vi "test_generic.vi"() -> ()   [LabVIEW 2017, in "GenericDAQ.lvclass"]
uses:
  GenericDAQ.lvclass
  Clock/GenericClock/GenericClock/GenericClock.lvclass
  common/classes/GenericComponent/GenericComponent/GenericComponent.lvclass
  main/labview_source/type_definitions/clusters/controls_refs.ctl
  common/classes/ErrorController/ErrorController/ErrorController.lvclass
  common/classes/GenericToplevelComponent/GenericToplevelComponent/common_trigger_enum.ctl
  common/classes/GenericToplevelComponent/GenericToplevelComponent/GenericToplevelComponent.lvclass
  main/labview_source/type_definitions/enumerations/run_mode_enum.ctl
panel:
  out "error handler loaded?":bool
  in  "toggleAcquisitionButton":bool
  in  "continuous?":bool
  in  "samples to read":i32=1000000000
  in  "frequency":dbl[unit]=40000.0
  in  "createClockButton":bool
  in  "createDAQButton":bool
  out "error out":errorcluster
  in  "stopProgramButton":bool
  # "Test Suite for GenericDAQ"
  # "How to use this Test Suite\n\n1. Choose DAQ compoment and select configuration. \n2. Create and send DAQ component.\n3. Choose Clock component and select configuration.\n4. Create Clock component.\n5. Start Clock."
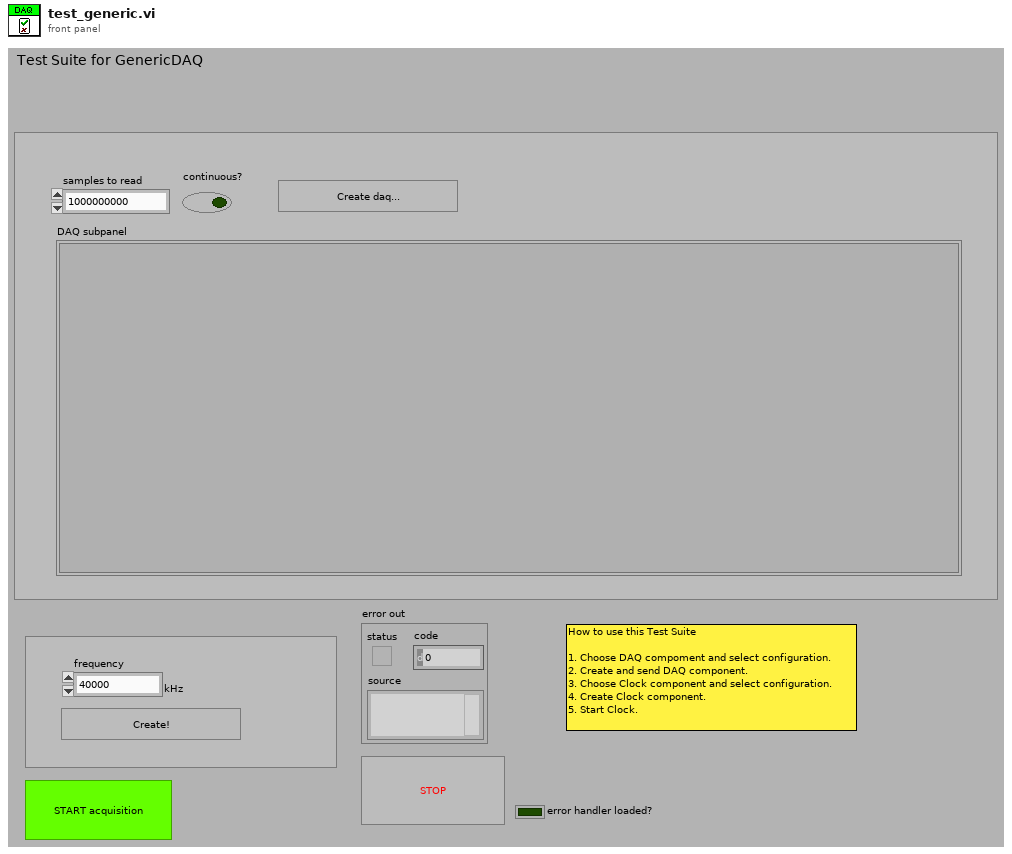
[diagram p1: front panel]
types:
  T1 = typedef "controls_refs.ctl" = cluster{"buttons":cluster{"start_focus":refnum<vi>, "start_single_sweep":refnum<vi>, "start_experiment":refnum<vi>, "save":refnum<vi>, "exit":refnum<vi>}, "tabs":cluster{"main":refnum<vi>, "settings":refnum<vi>}, "subpanels":cluster{"imagingMode":refnum<vi>, "scanHead":refnum<vi>, "display":refnum<vi>, "experimentController":refnum<vi>, "instrument":refnum<vi>, "stage":refnum<vi>, "stimulator":refnum<vi>, "dataCollection":refnum<vi>, "analyser":refnum<vi>, "daq":refnum<vi>, "imageAssembler":refnum<vi>}, "drop-downs":cluster{"imagingMode":refnum<vi>, "experimentalController":refnum<vi>, "objective":refnum<vi>}, "status lights":cluster{"experimentController":refnum<vi>, "imagingMode":refnum<vi>, "scanHead":refnum<vi>, "daq":refnum<vi>, "imageAssembler":refnum<vi>, "dataCollection":refnum<vi>, "display":refnum<vi>, "analyser":refnum<vi>, "stage":refnum<vi>, "stimulator":refnum<vi>, "instrument":refnum<vi>}, "message":refnum<vi>, "stimulator enabled?":refnum<vi>, "saving":cluster{"data folder path":refnum<vi>, "file base name":refnum<vi>, "notebook":refnum<vi>}, "progress bar":refnum<vi>, "update icon":refnum<vi>, "title":refnum<vi>, "main vi":refnum<vi>, "user":refnum<vi>}
  T2 = typedef "run_mode_enum.ctl" = enum16{"focus mode", "single sweep mode", "experiment mode"}
  T3 = typedef "GenericToplevelComponent.lvclass/common_trigger_enum.ctl" = enum16{"NULL", "initialise", "terminate", "fetch command", "fetch data", "attach observer", "register as observer", "detach observer", "acknowledge", "start", "stop", "sweep started", "sweep finished", "experiment started", "experiment stopped"}
  T4 = typedef "XComponentSpecification.xctl/data.ctl" = cluster{"class path":string, "configuration":string, "label":string, "settings name":string}
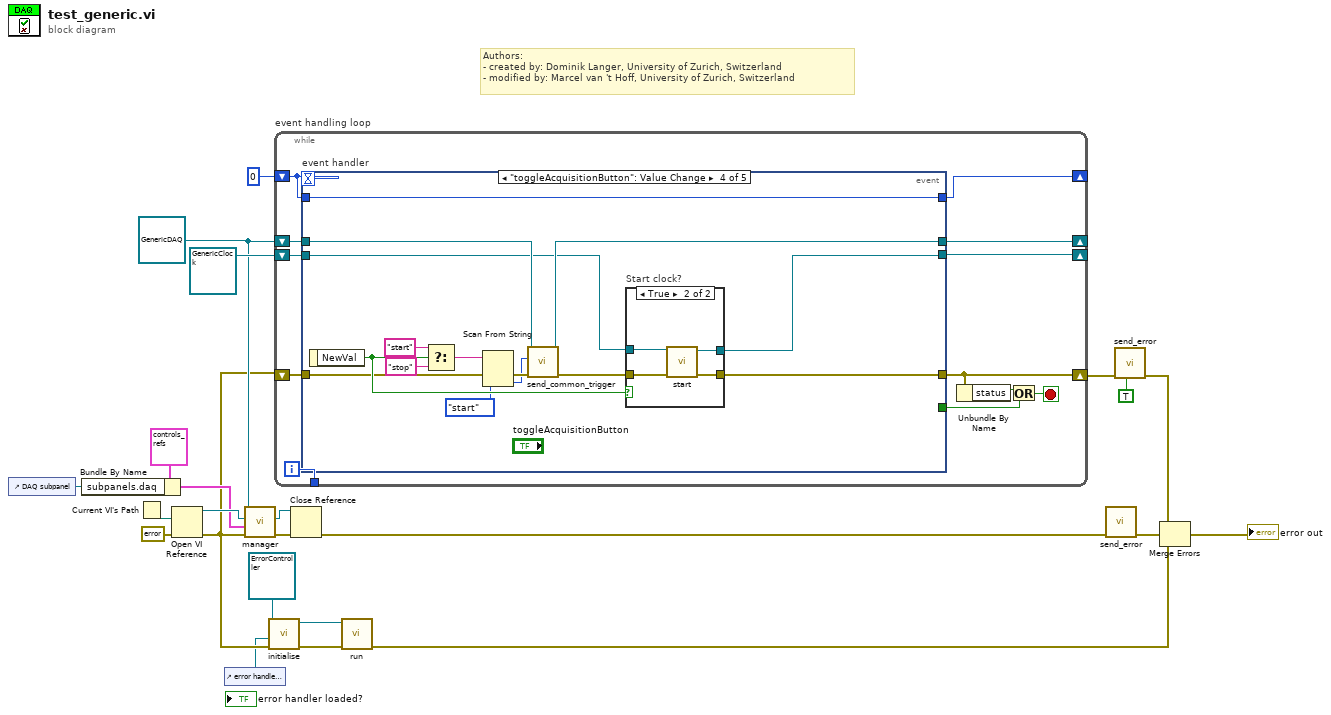
[diagram p0: block diagram]
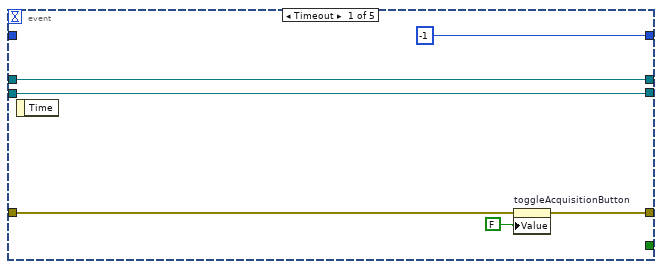
[diagram p2: hidden frame]
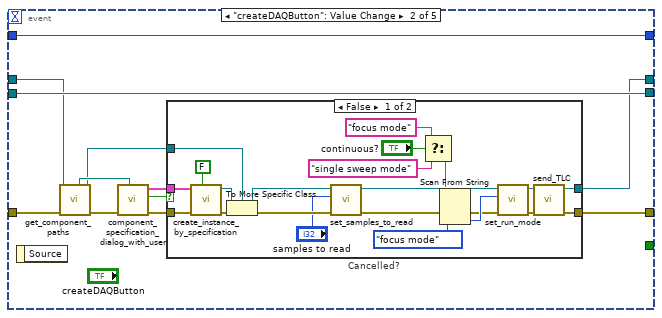
[diagram p3: hidden frame]
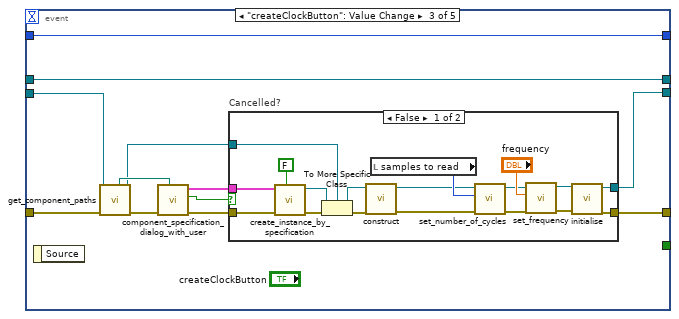
[diagram p5: hidden frame]
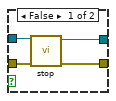
[diagram p7: hidden frame]
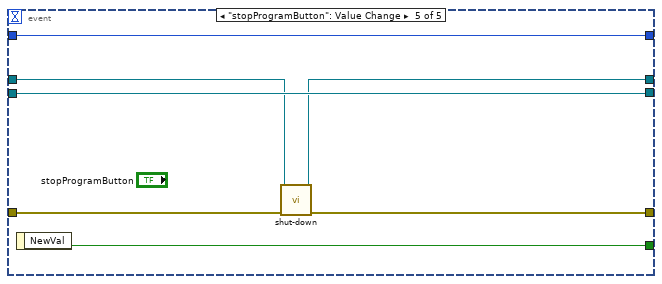
[diagram p8: hidden frame]
diagram:
  w12 = refnum<class "GenericDAQ.lvclass"> refnum ("GenericDAQ.lvclass")
  # "Authors: \n- created by: Dominik Langer, University of Zurich, Switzerland\n- modified by: Marcel van 't Hoff, University of Zurich, Switzerland"
  n1 = control-ref of="DAQ subpanel"() -> (w14:refnum<vi>)
  n2 = Bundle By Name(cluster=T1 {"buttons"={"start_focus"=refnum, "start_single_sweep"=refnum, "start_experiment"=refnum, "save"=refnum, "exit"=refnum}, "tabs"={"main"=refnum, "settings"=refnum}, "subpanels"={"imagingMode"=refnum, "scanHead"=refnum, "display"=refnum, "experimentController"=refnum, "instrument"=refnum, "stage"=refnum, "stimulator"=refnum, "dataCollection"=refnum, "analyser"=refnum, "daq"=refnum, "imageAssembler"=refnum}, "drop-downs"={"imagingMode"=refnum, "experimentalController"=refnum, "objective"=refnum}, "status lights"={"experimentController"=refnum, "imagingMode"=refnum, "scanHead"=refnum, "daq"=refnum, "imageAssembler"=refnum, "dataCollection"=refnum, "display"=refnum, "analyser"=refnum, "stage"=refnum, "stimulator"=refnum, "instrument"=refnum}, "message"=refnum, "stimulator enabled?"=refnum, "saving"={"data folder path"=refnum, "file base name"=refnum, "notebook"=refnum}, "progress bar"=refnum, "update icon"=refnum, "title"=refnum, "main vi"=refnum, "user"=refnum} ("control references"), "subpanels.daq"=w14) -> (w15:T1)
  n3 = Current VI's Path() -> (path=w20:path)
  n4 = Open VI Reference(vi path=w20, error in (no error)=errorcluster {"status"=FALSE, "code"=0, "source"=""}) -> (vi reference=w18:refnum<vi>, error out=w5:errorcluster)  [unwired: 4 in]
  n5 = control-ref of="error handler loaded?"() -> (w2:refnum<vi>)
  n6 = call-dynamic "manager.vi"("error in (no error)"=w5, "control references"=w15, "top-level VI ref in"=w18, "GenericToplevelComponent in"=w12) -> ("error out"=w17:errorcluster, "top-level VI ref out"=w13:refnum<vi>)  [unwired: 5 in, 1 out]
  n7 = call-dynamic "initialise.vi"("error in (no error)"=w5, "error boolean"=w2, "ErrorController in"=refnum<class "ErrorController.lvclass"> refnum) -> ("error out"=w4:errorcluster, "ErrorController out"=w3:refnum<class "ErrorController.lvclass">)  [unwired: 7 in]
  n8 = while "event handling loop" {
    shift-right: [w34] -> _
    shift-left: 0 -> [w35]
    shift-right: [w27] -> w11
    shift-left: w5 -> [w33]
    shift-right: [w31] -> _
    shift-left: w12 -> [w32]
    shift-right: [w29] -> _
    shift-left: refnum<class "GenericClock.lvclass"> refnum ("GenericClock.lvclass") -> [w30]
    tunnel: [w28] -> _
    i -> [w28]
    stop <- w25 stop-if-true
    n9 = event "event handler" shown="[3] \"toggleAcquisitionButton\": Value Change" {
      selector: _ -> [_ _ _ _ _]
      dyn-events: _ -> [_ _ _ _ _]
      timeout: w35 -> [_ _ _ _ _]
      tunnel: [-1 w53 w89 w124 w139] -> w34
      tunnel: w35 -> [_ w53 w89 w124 w139]
      tunnel: [w40 w51 w87 w120 w136] -> w27
      tunnel: w33 -> [w36 w47 w83 w116 w137]
      tunnel: [_ _ _ _ w133] -> w24
      tunnel: [w38 w50 w88 w122 w134] -> w31
      tunnel: w32 -> [w38 w44 w88 w123 w135]
      tunnel: [w37 w52 w86 w118 w138] -> w29
      tunnel: w30 -> [w37 w52 w81 w119 w138]
      event Timeout {
        n10 = event-data() -> ()  [unwired: 2 out]
        n11 = property on="toggleAcquisitionButton" class="Bool (strict)"(error in=w36, "Value"=FALSE ("toggleDAQButton")) -> (error out=w40:errorcluster)  [unwired: 1 in, 1 out]
      }
      event "createDAQButton": Value Change {
        n12 = event-data() -> ()  [unwired: 2 out]
        n13 = call-dynamic "get_component_paths.vi"("error in (no error)"=w47, "GenericComponent in"=w44) -> ("error out"=w48:errorcluster, "GenericComponent out"=w43:refnum<class "GenericDAQ.lvclass">, "component type directory"=w49:path)  [unwired: 4 in, 3 out]
        n14 = call "component_specification_dialog_with_user.vi"("start path"=w49, "error in (no error)"=w48) -> ("error out"=w46:errorcluster, "cancelled?"=w42:bool, "component specification out"=w45:T4)  [unwired: 7 in]
        n15 = case "Cancelled?" shown="False" w42 {
          tunnel: [w73 w77] -> w51
          tunnel: [w72 w76] -> w50
          tunnel: w46 -> [w63 w77]
          tunnel: w45 -> [w62 _]
          tunnel: w43 -> [w61 w76]
          frame False {
            n16 = call "create_instance_by_specification.vi"("call constructor?"=FALSE, "error in (no error)"=w63, "component specification"=w62) -> ("error out"=w75:errorcluster, "GenericPlugin out"=w74:refnum<class "GenericComponent.lvclass">)  [unwired: 6 in, 1 out]
            n17 = To More Specific Class(target class=w61, reference=w74, error in=w75) -> (specific class reference=w70:refnum<class "GenericDAQ.lvclass">, error out=w71:errorcluster)
            n18 = call-dynamic "set_samples_to_read.vi"("error in (no error)"=w71, "samples to read"="samples to read", "GenericDAQ.lvclass in"=w70) -> ("error out"=w56:errorcluster, "GenericDAQ.lvclass out"=w67:refnum<class "GenericDAQ.lvclass">)  [unwired: 7 in]
            n19 = Select(t="focus mode", s="continuous?", f="single sweep mode") -> (s? t:f=w58:string)
            n20 = Scan From String(input string=w58, error in=w56, default 1=run_mode_enum."focus mode" ("t")) -> (error out=w55:errorcluster, output 1=w57:T2)  [unwired: 2 in, 2 out]
            n21 = call-dynamic "set_run_mode.vi"("error in (no error)"=w55, "run mode"=w57, "GenericPlugin in"=w67) -> ("error out"=w68:errorcluster, "GenericPlugin out"=w66:refnum<class "GenericDAQ.lvclass">)  [unwired: 7 in]
            n22 = call-dynamic "send_TLC.vi"("error in (no error)"=w68, "GenericToplevelComponent in"=w66) -> ("error out"=w73:errorcluster, "GenericToplevelComponent out"=w72:refnum<class "GenericDAQ.lvclass">)  [unwired: 8 in]
          }
          frame True {
          }
        }
      }
      event "createClockButton": Value Change {
        n23 = event-data() -> ()  [unwired: 2 out]
        n24 = call-dynamic "get_component_paths.vi"("error in (no error)"=w83, "GenericComponent in"=w81) -> ("error out"=w85:errorcluster, "GenericComponent out"=w80:refnum<class "GenericClock.lvclass">, "component type directory"=w84:path)  [unwired: 4 in, 3 out]
        n25 = call "component_specification_dialog_with_user.vi"("start path"=w84, "error in (no error)"=w85) -> ("error out"=w82:errorcluster, "cancelled?"=w79:bool, "component specification out"=w78:T4)  [unwired: 7 in]
        n26 = case "Cancelled?" shown="False" w79 {
          tunnel: [w96 w109] -> w87
          tunnel: [w94 w108] -> w86
          tunnel: w82 -> [w92 w109]
          tunnel: w80 -> [w91 w108]
          tunnel: w78 -> [w90 _]
          frame False {
            n27 = call "create_instance_by_specification.vi"("call constructor?"=FALSE, "error in (no error)"=w92, "component specification"=w90) -> ("error out"=w107:errorcluster, "GenericPlugin out"=w106:refnum<class "GenericComponent.lvclass">)  [unwired: 6 in, 1 out]
            n28 = To More Specific Class(target class=w91, reference=w106, error in=w107) -> (specific class reference=w104:refnum<class "GenericClock.lvclass">, error out=w105:errorcluster)
            n29 = call-dynamic "construct.vi"("error in (no error)"=w105, "GenericPlugin in"=w104) -> ("error out"=w99:errorcluster, "GenericPlugin out"=w95:refnum<class "GenericClock.lvclass">)  [unwired: 8 in]
            n30 = local read "samples to read"() -> (w100:i32)
            n31 = call-dynamic "set_number_of_cycles.vi"("error in (no error)"=w99, "number of cycles"=w100, "GenericClock.lvclass in"=w95) -> ("error out"=w98:errorcluster, "GenericClock.lvclass out"=w102:refnum<class "GenericClock.lvclass">)  [unwired: 7 in]
            n32 = call-dynamic "set_frequency.vi"("error in (no error)"=w98, "frequency"="frequency", "GenericClock.lvclass in"=w102) -> ("error out"=w97:errorcluster, "GenericClock.lvclass out"=w101:refnum<class "GenericClock.lvclass">)  [unwired: 7 in]
            n33 = call-dynamic "initialise.vi"("error in (no error)"=w97, "GenericPlugin in"=w101) -> ("error out"=w96:errorcluster, "GenericPlugin out"=w94:refnum<class "GenericClock.lvclass">)  [unwired: 8 in]
          }
          frame True {
          }
        }
      }
      event "toggleAcquisitionButton": Value Change {
        n34 = event-data() -> ("NewVal"=w117:bool)  [unwired: 1 out]
        n35 = Select(t="start", s=w117, f="stop") -> (s? t:f=w111:string)
        n36 = Scan From String(input string=w111, error in=w116, default 1=common_trigger_enum."start" ("trigger")) -> (error out=w115:errorcluster, output 1=w110:T3)  [unwired: 2 in, 2 out]
        n37 = call-dynamic "send_common_trigger.vi"("error in (no error)"=w115, "trigger"=w110, "GenericToplevelComponent in"=w123) -> ("error out"=w121:errorcluster, "GenericToplevelComponent out"=w122:refnum<class "GenericDAQ.lvclass">)  [unwired: 6 in, 1 out]
        n38 = case "Start clock?" shown="True" w117 {
          tunnel: [w125 w132] -> w120
          tunnel: [w126 w131] -> w118
          tunnel: w121 -> [w128 w130]
          tunnel: w119 -> [w127 w129]
          frame False {
            n39 = call-dynamic "stop.vi"("error in (no error)"=w128, "GenericClock in"=w127) -> ("error out"=w125:errorcluster, "GenericClock out"=w126:refnum<class "GenericClock.lvclass">)  [unwired: 8 in]
          }
          frame True {
            n40 = call-dynamic "start.vi"("error in (no error)"=w130, "GenericClock in"=w129) -> ("error out"=w132:errorcluster, "GenericClock out"=w131:refnum<class "GenericClock.lvclass">)  [unwired: 8 in]
          }
        }
      }
      event "stopProgramButton": Value Change {
        n41 = event-data() -> ("NewVal"=w133:bool)  [unwired: 1 out]
        n42 = call-dynamic "shut-down.vi"("error in (no error)"=w137, "GenericToplevelComponent in"=w135) -> ("error out"=w136:errorcluster, "GenericToplevelComponent out"=w134:refnum<class "GenericDAQ.lvclass">)  [unwired: 8 in]
      }
    }
    n43 = Unbundle By Name(w27) -> ("status"=w26:bool)
    n44 = Or(x=w26, y=w24) -> (x .or. y?=w25:bool)
  }
  n45 = Close Reference(reference=w13, error in (no error)=w17) -> (error out=w8:errorcluster)
  n46 = call "run.vi"("error in (no error)"=w4, "ErrorController in"=w3) -> ("error out"=w1:errorcluster)  [unwired: 8 in, 1 out]
  n47 = call "send_error.vi"("error in (no error)"=w8) -> ("error out"=w7:errorcluster)  [unwired: 10 in]
  n48 = call "send_error.vi"("last error? (F)"=TRUE, "error in (no error)"=w11) -> ("error out"=w10:errorcluster)  [unwired: 9 in]
  n49 = Merge Errors(w10, w7, w1) -> (→"error out":errorcluster)
